vi "Set_PS2_0V.vi"(3 "error in":errorcluster) -> (10 "error out":errorcluster)   [LabVIEW 2015]
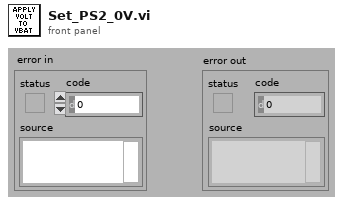
[diagram p1: front panel]
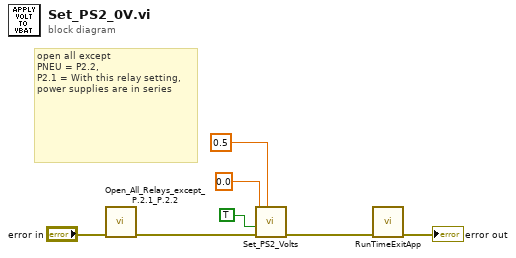
[diagram p0: block diagram]
diagram:
  # "open all except \nPNEU = P2.2, \nP2.1 = With this relay setting, power supplies are in series"
  n1 = call "Open_All_Relays_except_P.2.1_P.2.2.vi"("error in"="error in") -> ("error out"=w5:errorcluster)  [unwired: 9 in]
  n2 = call "Set_PS2_Volts.vi"("delay (secs)"=0.5, "error in"=w5, "Output on/off"=TRUE, "Output Voltage"=0.0) -> ("error out"=w4:errorcluster)  [unwired: 5 in, 2 out]
  n3 = call "RunTimeExitApp.vi"("error in (no error)"=w4) -> ("error out"=→"error out":errorcluster)  [unwired: 10 in]
